vi "Telescope Stop.vi"(8 "error in (no error)":errorcluster, 11 "PRIME Telescope in":refnum<class "PRIME Telescope.lvclass">) -> (0 "error out":errorcluster, 3 "PRIME Telescope out":refnum<class "PRIME Telescope.lvclass">)   [LabVIEW 2021, in "PRIME Telescope.lvclass"]
uses:
  PRIME Telescope.lvclass
  PRIME Telescope.lvclass/PRIME Telescope.ctl
  Telescope.lvclass
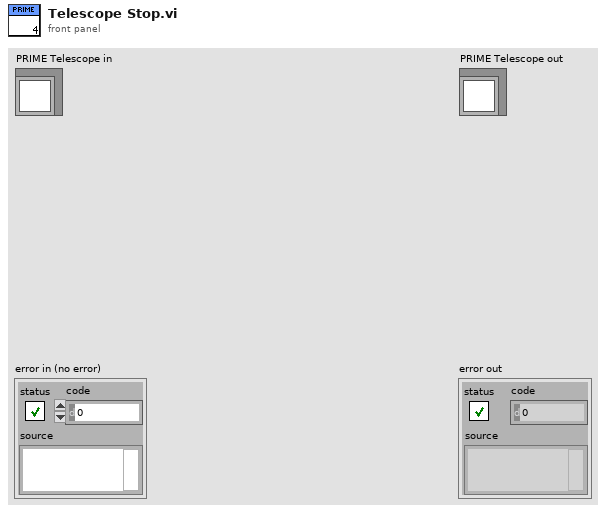
[diagram p1: front panel]
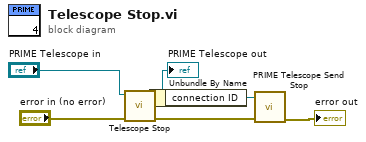
[diagram p0: block diagram]
diagram:
  n1 = call-parent "Telescope Stop.vi"("error in (no error)"="error in (no error)", "Telescope in"="PRIME Telescope in") -> ("error out"=w4:errorcluster, "Telescope out"=w2:refnum<class "PRIME Telescope.lvclass">)  [unwired: 8 in]
  "PRIME Telescope out" <- w2
  n2 = Unbundle By Name(w2) -> ("connection ID"=w1:refnum<k5>)
  n3 = call "PRIME Telescope Send Stop.vi"("error in (no error)"=w4, "connection ID"=w1) -> ("error out"=→"error out":errorcluster)  [unwired: 9 in]
